vi "Tile Picture by Row and Col.vi"(6 "Rows and Cols":i32[](array[numeric]), 7 "Start Point":cluster{"x":i16, "y":i16} caption="Start (x,y)", 8 "错误输入":errorcluster, 9 "Para":T2={"Frame?"=FALSE, "Pen and Color"={"pen"={"Width"=1, "Style"=enum."Solid"}, "color(black)"=0}}, 10 "image data":T1 caption="图像数据", 11 "Picture in":picture) -> (0 "错误输出":errorcluster, 3 "Picture out":picture)   [LabVIEW 2012, in "Picture Box Tools.lvlib"]
uses:
  Picture Box Tools.lvlib
  <vilib>/picture/picture.llb/imagedata.ctl
  Rectangle Tools/Rect/OffsetRect/OffsetRect by Point and Rect.vi
  Rectangle Tools/Rect/Rect Tools.lvlib
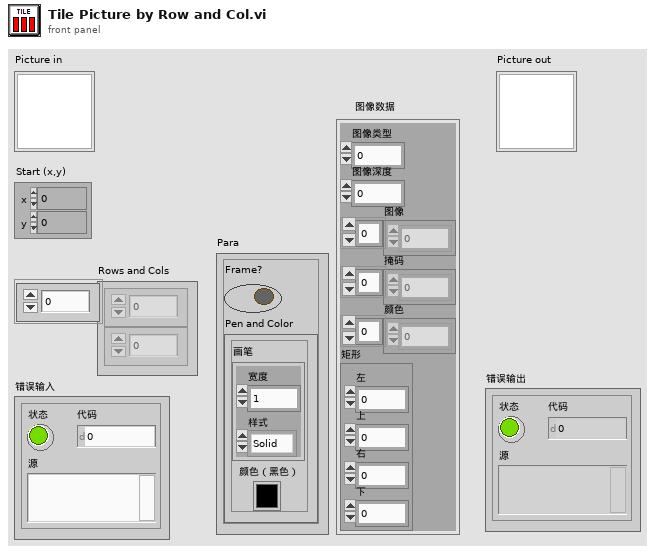
[diagram p1: front panel]
types:
  T1 = typedef "imagedata.ctl" = cluster{"image type":i32, "image depth":i32, "image":u8[], "mask":u8[], "colors":u32[], "Rectangle":cluster{"left":i16, "top":i16, "right":i16, "bottom":i16}}
  T2 = cluster{"Frame?":bool, "Pen and Color":cluster{"pen":cluster{"Width":i16, "Style":enum32{"Solid", "Dash", "Dot", "DashDot", "DashDotDot"}}, "color(black)":u32}}
  T3 = cluster{"pen":cluster{"Width":i16, "Style":enum32{"Solid", "Dash", "Dot", "DashDot", "DashDotDot"}}, "color(black)":u32}
  T4 = cluster{"left":i16, "top":i16, "right":i16, "bottom":i16}
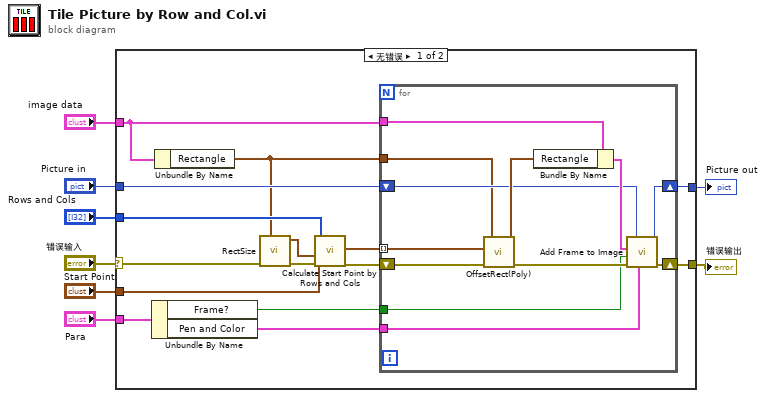
[diagram p0: block diagram]
diagram:
  n1 = case shown="无错误" "错误输入" {
    selector: "错误输入" -> [w11 w37]
    tunnel: [w14 w37] -> w7
    tunnel: "Picture in" -> [w13 w36]
    tunnel: [w15 w36] -> w5
    tunnel: "Para" -> [w23 _]
    tunnel: "image data" -> [w17 _]
    tunnel: "Rows and Cols" -> [w22 _]
    tunnel: "Start Point" -> [w21 _]
    frame No Error {
      n2 = Unbundle By Name(w23) -> ("Frame?"=w12:bool, "Pen and Color"=w16:T3)
      n3 = Unbundle By Name(w17) -> ("Rectangle"=w9:T4)
      n4 = call "RectSize.vi"("错误输入"=w11, "rect"=w9) -> ("错误输出"=w10:errorcluster, "point"=w20:cluster{"x":i16, "y":i16})  [unwired: 6 in, 2 out]
      n5 = call "Calculate Start Point by Rows and Cols.vi"("错误输入"=w10, "Size"=w20, "Start Point"=w21, "Rows and Cols"=w22) -> ("错误输出"=w18:errorcluster, "Start Point Array"=w19:cluster{"x":i16, "y":i16}[])  [unwired: 6 in]
      n6 = for {
        tunnel: w19 -> [w35] mode=indexing
        shift-right: [w28] -> w14
        shift-left: w18 -> [w34]
        shift-right: [w27] -> w15
        shift-left: w13 -> [w30]
        tunnel: w16 -> [w26]
        tunnel: w12 -> [w25]
        tunnel: w17 -> [w33]
        tunnel: w9 -> [w24]
        n7 = call-poly "OffsetRect(Poly).vi"("错误输入"=w34, "point"=w35, "rect"=w24) -> ("错误输出"=w29:errorcluster, "offset rect"=w32:T4)  [unwired: 7 in]
        n8 = Bundle By Name(cluster=w33, "Rectangle"=w32) -> (w31:T1)
        n9 = call "Add Frame to Image.vi"("Option"=w26, "错误输入"=w29, "Frame?"=w25, "image data"=w31, "Picture in"=w30) -> ("错误输出"=w28:errorcluster, "Picture out"=w27:picture)  [unwired: 5 in]
      }
    }
    frame Error {
    }
  }
  "Picture out" <- w5
  "错误输出" <- w7
